vi "Rectangular Target - 2013.vi"(9 "Original Image 2":T2(plugin-control)) -> (1 "data":T1)   [LabVIEW 2012]
doc: "This VI demonstrates how to do target processing on a laptop computer. It uses the same MJPG VI as the dashboard, sets a few of the important camera properties that impact processing, and carries out the same processing steps as the RT example also included in this project."
uses:
  TargetData.ctl
  <vilib>/vision/NI_Vision_Development_Module.lvlib
panel:
  in  "Camera Type":enum16{"206", "1011"}(ring)
  out "Target Info":T3(array[cluster])
  in  "Area Size Limit %":dbl=0.5
  in  "Particle Count Limit":i32=10
  in  "Score Limits":T4={"Rect Coverage"=60.0, "X Edge Strength"=40.0, "Y Edge Strength"=60.0, "Center"=75.0, "Outer"=75.0}
  in  "Processing":enum32{"Color", "Monochrome"}(tab)
  out "Value":cluster{i32, i32}
  out "Saturation":cluster{i32, i32}
  in  "Value":i32=120
  in  "Saturation":i32=200
  in  "Hue":i32(knob)=79 scale=0.0..255.0
  in  "Margins":cluster{"Hue":i32, "Sat":i32, "Val":i32}={"Hue"=29, "Sat"=80, "Val"=80} {"Sat" scale=0.0..80.0; "Val" scale=0.0..80.0; "Hue" scale=0.0..80.0}
  out "Hue":cluster{i32, i32}
  in  "Range":cluster{"Lower value":sgl, "Upper value":sgl}={"Lower value"=150.0, "Upper value"=255.0} {"Lower value" scale=0.0..255.0; "Upper value" scale=0.0..255.0}
  in  "Color Plane":i32(ring)=6 items=["Red", "Green", "Blue", "Hue", "Saturation", "Luminance", "Value", "Intensity"]
  in  "Annotate":bool=TRUE
  out "Processed Image":T2(plugin-control)
  out "Original Image":T2(plugin-control)
  # "Information:\nProcessing can be based on color or light intensity.\nParticles within the image are scored by rectangle coverage, aspect ratio, and\nedge strength/hollowness. A particle is considered a target if all scores\nare above the score limits you set. Particles can be annotated -- surrounded by\na rectangle and scores drawn to the left .\nTo control the number of particles being scored, use the count limit and the size\nlimit.\nBe sure to set the Camera IP before running. The distance calculation uses the\ncamera type to index the value of the lens view angle."
  # "Click in the image to choose  color for processing."
  # "Green scores are above the limit, orange are below. Inner/outer rect\nindicates all passed."
  # "Lower/Upper"
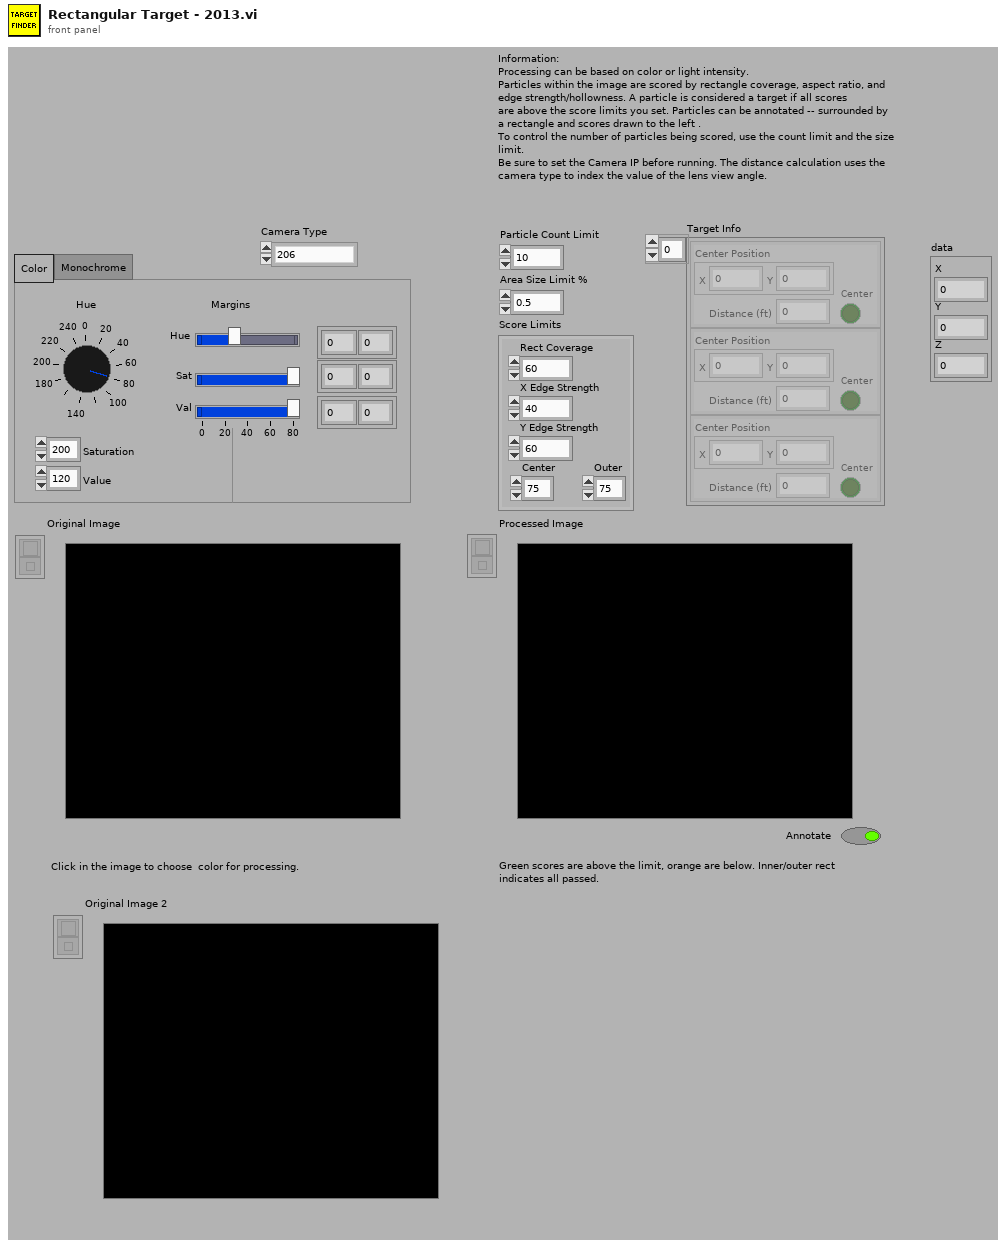
[diagram p1: front panel]
types:
  T1 = typedef "TargetData.ctl" = cluster{"X":dbl, "Y":dbl, "Z":dbl}
  T2 = typedef "IMAQ Image.ctl" = refnum<image>
  T3 = cluster{"Center Position":cluster{"X":dbl, "Y":dbl}, "Distance (ft)":dbl, "Center":bool}[]
  T4 = cluster{"Rect Coverage":dbl, "X Edge Strength":dbl, "Y Edge Strength":dbl, "Center":dbl, "Outer":dbl}
  T5 = cluster{"Position":cluster{"X":dbl, "Y":dbl}, "Distance (ft)":dbl, bool}[]
  T6 = typedef "Image Type" = u32
  T7 = cluster{cluster{"Left":dbl, "Top":dbl, "Right":dbl, "Bottom":dbl}, "Scores":dbl[], cluster{"Long":dbl, "Short":dbl}}[]
  T8 = cluster{"Target Center (-1 to 1)":cluster{"X":dbl, "Y":dbl}, "Distance (ft)":dbl, "Center Target":bool}
  T9 = cluster{"Target Center (-1 to 1)":cluster{"X":dbl, "Y":dbl}, "Distance (ft)":dbl, "Center Target":bool}[]
  T10 = cluster{"Position":cluster{"X":dbl, "Y":dbl}, "Distance (ft)":dbl, bool}
  T11 = cluster{"Left":dbl, "Top":dbl, "Right":dbl, "Bottom":dbl}
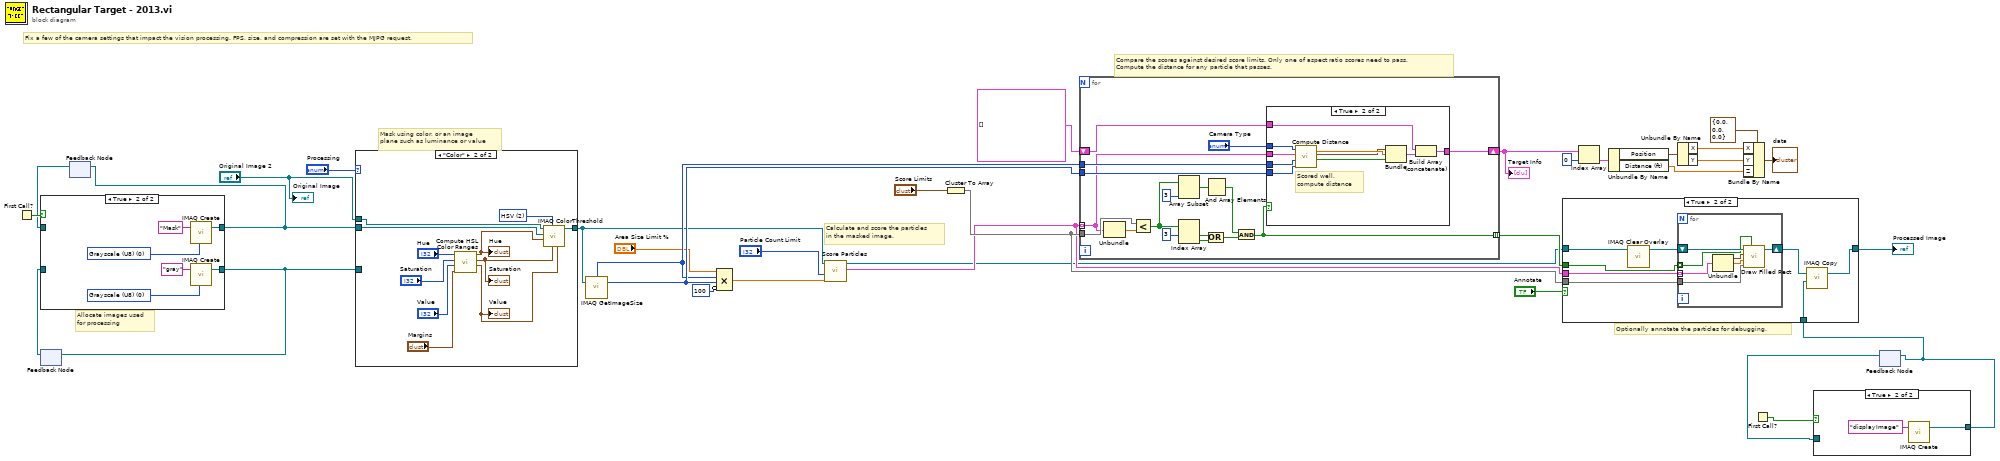
[diagram p0: block diagram]
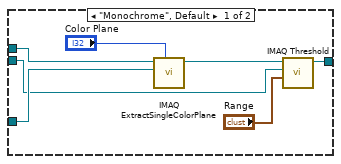
[diagram p5: hidden frame]
diagram:
  # "Optionally annotate the particles for debugging."
  # "Compare the scores against desired score limits. Only one of aspect ratio scores need to pass.\nCompute the distance for any particle that passes."
  # "Calculate and score the particles\nin the masked image."
  # "Mask using color, or an image\nplane such as luminance or value"
  # "Allocate images used\nfor processing"
  # "Fix a few of the camera settings that impact the vision processing. FPS, size, and compression are set with the MJPG request."
  n1 = First Call?() -> (First Call?: T/F=w8:bool)
  n2 = feedback #1() -> (w4:T2)  [unwired: 1 in]
  n3 = feedback #2() -> (w5:T2)  [unwired: 1 in]
  n4 = case shown="True" w8 {
    tunnel: [w35 w37] -> w7
    tunnel: [w36 w38] -> w6
    tunnel: w5 -> [w36 _]
    tunnel: w4 -> [w35 _]
    frame False {
    }
    frame True {
      w42 = T6 0 items=["Grayscale (U8)", "Grayscale (I16)", "Grayscale (SGL)", "Complex (CSG)", "RGB (U32)", "HSL (U32)", "RGB (U64)", "Grayscale (U16)"] ("Image Type")
      w39 = T6 0 items=["Grayscale (U8)", "Grayscale (I16)", "Grayscale (SGL)", "Complex (CSG)", "RGB (U32)", "HSL (U32)", "RGB (U64)", "Grayscale (U16)"] ("Image Type")
      n5 = call "IMAQ Create"("Image Name"="Mask", "Image Type"=w42) -> ("New Image"=w38:T2)  [unwired: 2 in, 2 out]
      n6 = call "IMAQ Create"("Image Name"="gray", "Image Type"=w39) -> ("New Image"=w37:T2)  [unwired: 2 in, 2 out]
    }
  }
  n7 = feedback-in #1(w7) -> ()
  n8 = feedback-in #2(w6) -> ()
  n9 = case shown="\"Color\"" "Processing" {
    tunnel: "Original Image 2" -> [w49 w60]
    tunnel: w7 -> [w48 _]
    tunnel: [w45 w59] -> w24
    tunnel: w6 -> [w43 w50]
    frame "Monochrome", Default {
      n10 = call "IMAQ ExtractSingleColorPlane"("Color Plane"="Color Plane", "Image Dst"=w48, "Image Src"=w49) -> ("Image Dst Out"=w47:T2)  [unwired: 1 in, 7 out]
      n11 = call "IMAQ Threshold"("Range"="Range", "Image Dst"=w43, "Image Src"=w47) -> ("Image Dst Out"=w45:T2)  [unwired: 3 in, 5 out]
    }
    frame "Color" {
      w58 = u16 2 items=["RGB", "HSL", "HSV", "HSI"] ("Color Mode")
      n12 = call "Compute HSL Color Ranges.vi"("Margins"="Margins", "Luminance"="Value", "Saturation"="Saturation", "Hue"="Hue") -> ("Lum Range"=w51:cluster{i32, i32}, "Sat Range"=w52:cluster{i32, i32}, "Hue Range"=w57:cluster{i32, i32})  [unwired: 5 in]
      "Hue" <- w57
      "Saturation" <- w52
      "Value" <- w51
      n13 = call "IMAQ ColorThreshold"("Blue or Luma or Val or Inten Range"=w51, "Green or Sat Range"=w52, "Color Mode"=w58, "Red or Hue Range"=w57, "Image Dst"=w50, "Image Src"=w60) -> ("Image Dst Out"=w59:T2)  [unwired: 4 in, 1 out]
    }
  }
  n14 = call "IMAQ GetImageSize"("Image"=w24) -> ("Y Resolution"=w31:i32, "X Resolution"=w30:i32)  [unwired: 3 in, 1 out]
  n15 = Compound Arithmetic op=MULTIPLY("Area Size Limit %", w30, w31, invert 100 ("value")) -> (w32:dbl)
  n16 = call "Score Particles.vi"("Area Size Limit"=w32, "Particle Count Limit"="Particle Count Limit", "Image Refnum in"=w24) -> ("Scored Particle Info"=w22:T7, "Image Refnum out"=w19:T2)  [unwired: 7 in]
  n17 = Cluster To Array(cluster="Score Limits") -> (array=w27:dbl[])
  n18 = for {
    shift-right: [w76] -> w16
    shift-left: T5 [] -> [w77]
    tunnel: w30 -> [w75]
    tunnel: w22 -> [w61] mode=indexing
    tunnel: w27 -> [w73]
    tunnel: w31 -> [w72]
    tunnel: [w63] -> w28 mode=indexing
    n19 = Unbundle(w61) -> ("Scores"=w74:dbl[])  [unwired: 2 out]
    n20 = Less?(x=w73, y=w74) -> (x < y?=w69:bool[])
    n21 = Array Subset(array=w69, length=3) -> (w70:bool[])  [unwired: 1 in]
    n22 = Index Array(array=w69, index #1=3 ("length")) -> (element #1=w67:bool, element #2=w66:bool)  [unwired: 1 in]
    n23 = Or(x=w67, y=w66) -> (x .or. y?=w65:bool)
    n24 = And Array Elements(Boolean array=w70) -> (logical AND=w64:bool)
    n25 = And(x=w64, y=w65) -> (x .and. y?=w63:bool)
    n26 = case shown="True" w63 {
      tunnel: w77 -> [w78 w88]
      tunnel: [w78 w87] -> w76
      tunnel: w75 -> [_ w85]
      tunnel: "Camera Type" -> [_ w83]
      tunnel: w72 -> [_ w81]
      tunnel: w61 -> [_ w80]
      frame False {
        # "Didn't score well enough"
      }
      frame True {
        # "Scored well,\ncompute distance"
        n27 = call "Compute Distance.vi"("Y Image Resolution"=w81, "X Image Resolution"=w85, "Particle Scores"=w80, "Camera Type"=w83) -> ("Center Target"=w79:bool, "Target Center (-1 to 1)"=w82:cluster{"X":dbl, "Y":dbl}, "Distance (ft)"=w84:dbl)  [unwired: 5 in]
        n28 = Bundle("Target Center (-1 to 1)"=w82, "Distance (ft)"=w84, "Center Target"=w79) -> (w86:T8)  [unwired: 1 in]
        n29 = Build Array (concatenate)(w88, w86) -> (w87:T9)
      }
    }
  }
  "Target Info" <- w16
  n30 = Index Array(array=w16, index=0) -> (element=w15:T10)
  n31 = Unbundle By Name(w15) -> ("Position"=w14:cluster{"X":dbl, "Y":dbl}, "Distance (ft)"=w11:dbl)
  n32 = Unbundle By Name(w14) -> ("X"=w13:dbl, "Y"=w12:dbl)
  n33 = Bundle By Name(cluster=T1 {"X"=0.0, "Y"=0.0, "Z"=0.0}, "X"=w13, "Y"=w12, "Z"=w11) -> (→"data":T1)
  n34 = First Call?() -> (First Call?: T/F=w3:bool)
  n35 = feedback #3() -> (w2:T2)  [unwired: 1 in]
  n36 = case shown="True" w3 {
    tunnel: [w89 w90] -> w1
    tunnel: w2 -> [w89 _]
    frame False {
    }
    frame True {
      n37 = call "IMAQ Create"("Image Name"="displayImage") -> ("New Image"=w90:T2)  [unwired: 4 in, 1 out]
    }
  }
  n38 = case shown="True" "Annotate" {
    tunnel: w19 -> [w92 w100]
    tunnel: [w92 w93] -> w21
    tunnel: w22 -> [_ w98]
    tunnel: w27 -> [_ w97]
    tunnel: w28 -> [_ w96]
    tunnel: w1 -> [_ w94]
    frame False {
    }
    frame True {
      n39 = call "IMAQ Clear Overlay"("Image"=w100) -> ("Image Out"=w99:T2)  [unwired: 2 in, 8 out]
      n40 = for {
        shift-right: [w106] -> w95
        shift-left: w99 -> [w107]
        tunnel: w98 -> [w103] mode=indexing
        tunnel: w97 -> [w102]
        tunnel: w96 -> [w101] mode=indexing
        n41 = Unbundle(w103) -> (w104:T11, "Scores"=w105:dbl[])  [unwired: 1 out]
        n42 = call "Draw Filled Rect.vi"("Limit Passed"=w101, "Limits"=w102, "Scores"=w105, "Bounding Box"=w104, "image in"=w107) -> ("image out"=w106:T2)  [unwired: 6 in]
      }
      n43 = call "IMAQ Copy"("Image Dst"=w94, "Image Src"=w95) -> ("Image Dst Out"=w93:T2)  [unwired: 4 in, 1 out]
    }
  }
  "Processed Image" <- w21
  n44 = feedback-in #3(w1) -> ()
  "Original Image" <- "Original Image 2"
